vi "DelayGeneratorController.vi"() -> ()   [LabVIEW 2009, in "DelayGenerator.lvlib"]
uses:
  DelayGenerator.lvlib
  Controls/DelayGeneratorState.ctl
  Aerotech/Controls/AerotechTarget.ctl
  Controls/DelayGeneratorCommand.ctl
panel:
  out "Target":T1
  out "State":T2
  in  "PROCESS":string="DELAYGENERATOR"
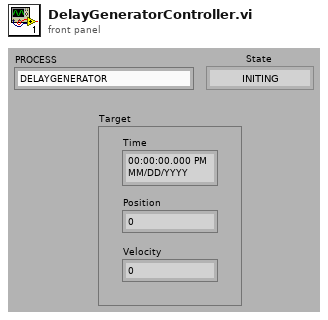
[diagram p1: front panel]
types:
  T1 = typedef "AerotechTarget.ctl" = cluster{"Time":timestamp, "Position":dbl, "Velocity":dbl}
  T2 = typedef "DelayGeneratorState.ctl" = enum16{"INITING", "IDLING", "TRACKING", "STOPPING"}
  T3 = typedef "DelayGeneratorCommand.ctl" = enum16{"IDLE", "TRACK", "QUIT"}
  T4 = typedef "DelayGeneratorSynchro.ctl" = cluster{"Command":refnum<queue>, "State":refnum<notifier>, "Offset":refnum<notifier>, "AerotechTarget":refnum<notifier>}
  T5 = typedef "DelayTarget.ctl" = cluster{"Time":timestamp, "Position":dbl[unit], "Velocity":dbl[unit]}
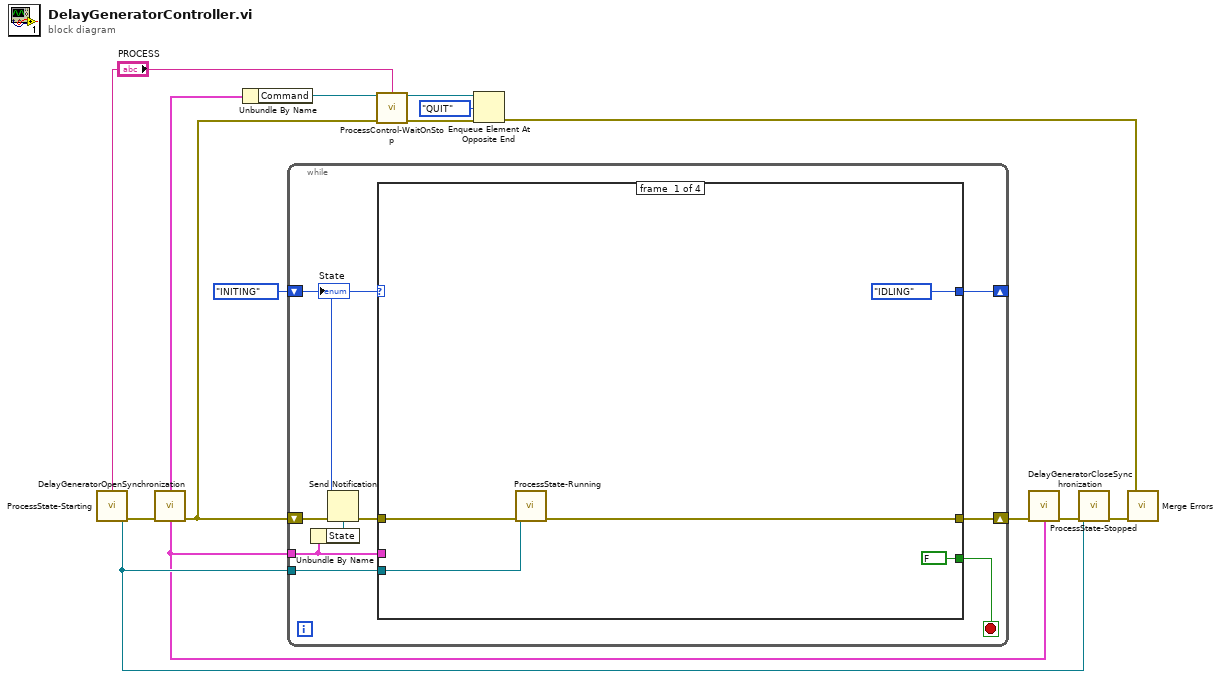
[diagram p0: block diagram]
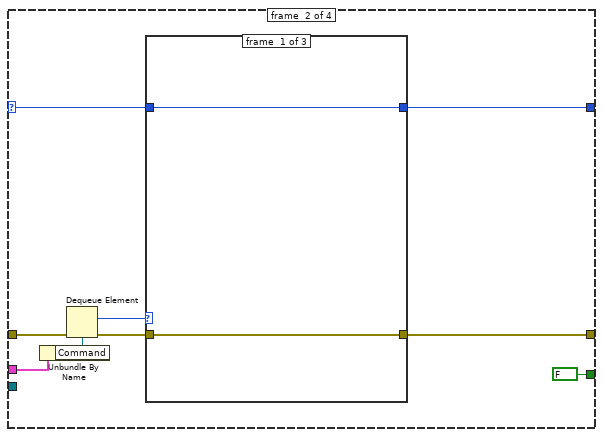
[diagram p2: hidden frame]
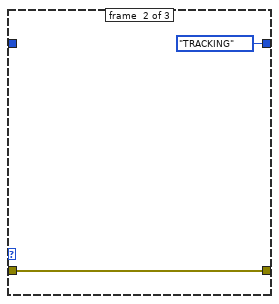
[diagram p3: hidden frame]
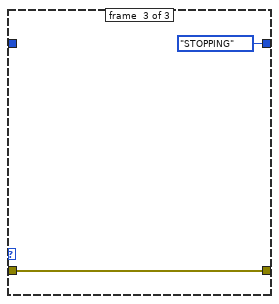
[diagram p4: hidden frame]
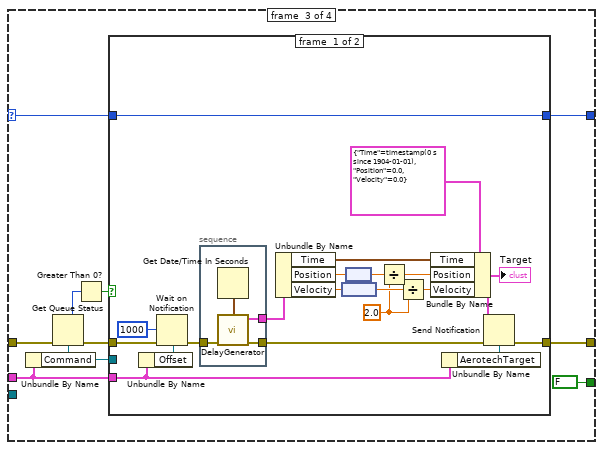
[diagram p5: hidden frame]
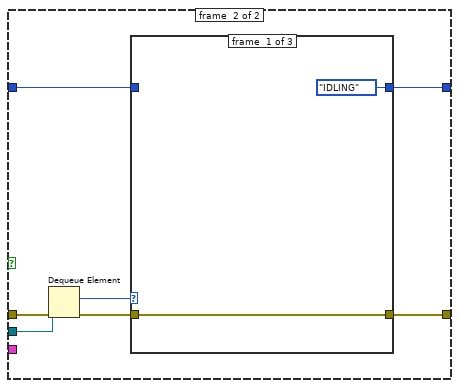
[diagram p6: hidden frame]
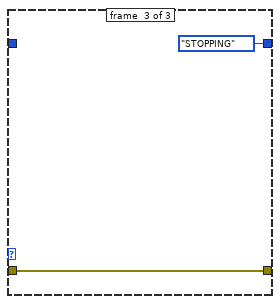
[diagram p8: hidden frame]
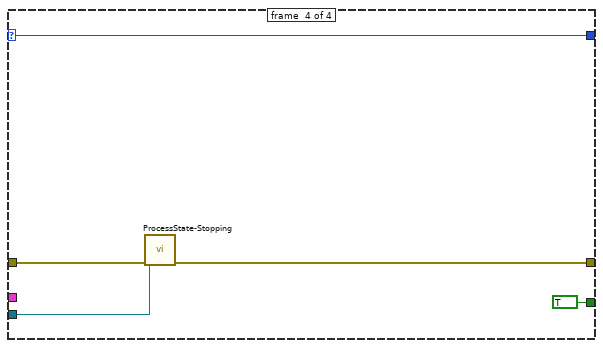
[diagram p9: hidden frame]
diagram:
  n1 = call "ProcessState-Starting.vi"("PROCESS"="PROCESS") -> ("ProcessStateNotifier"=w4:refnum<notifier>, "error in (no error)"=w13:errorcluster)  [unwired: 7 in]
  n2 = call "DelayGeneratorOpenSynchronization.vi"("error in (no error)"=w13) -> ("Synchro"=w1:T4, "error out"=w12:errorcluster)  [unwired: 7 in]
  n3 = Unbundle By Name(w1) -> ("Command"=w10:refnum<queue>)
  n4 = while {
    shift-right: [w15] -> w3
    shift-left: w12 -> [w19]
    shift-right: [w21] -> _
    shift-left: DelayGeneratorState."INITING" ("DelayGeneratorState") -> [w17]
    tunnel: w1 -> [w20]
    tunnel: w4 -> [w14]
    stop <- w22 stop-if-true
    n5 = Unbundle By Name(w20) -> ("State"=w18:refnum<notifier>)
    n6 = Send Notification(notification=w17, notifier=w18, error in (no error)=w19) -> (error out=w16:errorcluster)  [unwired: 1 out]
    n7 = case shown="\"TRACKING\"" w17 {
      selector: w17 -> [_ w31 w49 w93]
      tunnel: w16 -> [w26 w35 w52 w92]
      tunnel: w20 -> [_ w36 w46 _]
      tunnel: [FALSE FALSE FALSE TRUE] -> w22
      tunnel: [DelayGeneratorState."IDLING" ("DelayGeneratorState") w30 w44 w93] -> w21
      tunnel: [w25 w28 w43 w91] -> w15
      tunnel: w14 -> [w24 _ _ w90]
      frame #0 {
        n8 = call "ProcessState-Running.vi"("ProcessStateNotifier in"=w24, "error in (no error)"=w26) -> ("error out"=w25:errorcluster)  [unwired: 6 in, 1 out]
      }
      frame #1 {
        n9 = Unbundle By Name(w36) -> ("Command"=w34:refnum<queue>)
        n10 = Dequeue Element(queue=w34, error in (no error)=w35) -> (element=w33:T3, error out=w32:errorcluster)  [unwired: 1 in, 2 out]
        n11 = case shown="\"TRACK\"" w33 {
          tunnel: w32 -> [w38 w39 w42]
          tunnel: [w38 w39 w42] -> w28
          tunnel: w31 -> [w37 _ _]
          tunnel: [w37 DelayGeneratorState."TRACKING" ("DelayGeneratorState") DelayGeneratorState."STOPPING" ("DelayGeneratorState")] -> w30
          frame #0 {
          }
          frame #1 {
          }
          frame #2 {
          }
        }
      }
      frame #2 {
        n12 = Unbundle By Name(w46) -> ("Command"=w45:refnum<queue>)
        n13 = Get Queue Status(queue=w45, error in (no error)=w52) -> (error out=w48:errorcluster, # elements in queue=w51:i32)  [unwired: 1 in, 6 out]
        n14 = Greater Than 0?(x=w51) -> (x > 0?=w47:bool)
        n15 = case shown="False" w47 {
          tunnel: w49 -> [w58 w80]
          tunnel: w48 -> [w72 w83]
          tunnel: w46 -> [w68 _]
          tunnel: [w66 w78] -> w43
          tunnel: w45 -> [_ w82]
          tunnel: [w58 w79] -> w44
          frame #0 {
            w53 = 2.0 ("y")
            n16 = Unbundle By Name(w68) -> ("Offset"=w71:refnum<notifier>)
            n17 = Wait on Notification(notifier=w71, timeout in ms (-1)=1000, error in (no error)=w72) -> (error out=w69:errorcluster)  [unwired: 1 in, 3 out]
            n18 = stacked-sequence {
              tunnel: w69 -> [w76]
              tunnel: [w74] -> w67
              tunnel: [w73] -> w64
              frame #0 {
                n19 = Get Date/Time In Seconds() -> (seconds since 1Jan1904=w75:timestamp)
                n20 = call "DelayGenerator.vi"("error in (no error)"=w76, "Time Stamp"=w75) -> ("error out"=w74:errorcluster, "DelayTarget"=w73:T5)  [unwired: 8 in]
              }
            }
            n21 = Unbundle By Name(w64) -> ("Time"=w62:timestamp, "Position"=w60:dbl[unit], "Velocity"=w59:dbl[unit])
            n22 = node(w59) -> (w56:dbl)
            n23 = node(w60) -> (w55:dbl)
            n24 = Divide(x=w55, y=w53) -> (x/y=w57:dbl)
            n25 = Divide(x=w56, y=w53) -> (x/y=w54:dbl)
            n26 = Bundle By Name(cluster=T1 {"Time"=timestamp(0 s since 1904-01-01), "Position"=0.0, "Velocity"=0.0} ("notification"), "Time"=w62, "Position"=w57, "Velocity"=w54) -> (w61:T1)
            "Target" <- w61
            n27 = Unbundle By Name(w68) -> ("AerotechTarget"=w65:refnum<notifier>)
            n28 = Send Notification(notification=w61, notifier=w65, error in (no error)=w67) -> (error out=w66:errorcluster)  [unwired: 1 out]
          }
          frame #1 {
            n29 = Dequeue Element(queue=w82, error in (no error)=w83) -> (element=w81:T3, error out=w77:errorcluster)  [unwired: 1 in, 2 out]
            n30 = case shown="\"TRACK\"" w81 {
              tunnel: w80 -> [_ w87 _]
              tunnel: [DelayGeneratorState."IDLING" ("DelayGeneratorState") w87 DelayGeneratorState."STOPPING" ("DelayGeneratorState")] -> w79
              tunnel: [w84 w86 w88] -> w78
              tunnel: w77 -> [w84 w86 w88]
              frame #0 {
              }
              frame #1 {
              }
              frame #2 {
              }
            }
          }
        }
      }
      frame #3 {
        n31 = call "ProcessState-Stopping.vi"("ProcessStateNotifier in"=w90, "error in (no error)"=w92) -> ("error out"=w91:errorcluster)  [unwired: 6 in, 1 out]
      }
    }
    "State" <- w17
  }
  n32 = call "ProcessControl-WaitOnStop.vi"("PROCESS"="PROCESS", "error out"=w12) -> ("error in"=w11:errorcluster)  [unwired: 7 in]
  n33 = Enqueue Element At Opposite End(queue=w10, element=DelayGeneratorCommand."QUIT", error in (no error)=w11) -> (error out=w7:errorcluster)  [unwired: 1 in, 2 out]
  n34 = call "DelayGeneratorCloseSynchronization.vi"("Synchro"=w1, "error in (no error)"=w3) -> ("error out"=w2:errorcluster)  [unwired: 7 in]
  n35 = call "ProcessState-Stopped.vi"("ProcessStateNotifier in"=w4, "error in (no error)"=w2) -> ("error out"=w5:errorcluster)  [unwired: 7 in]
  n36 = call <vilib>:"Merge Errors.vi"("error in 3 (no error)"=w5, "error in 1 (no error)"=w7) -> ()  [unwired: 5 in, 1 out]
